vi "execute log.vi"(1 "log window":string, 2 "input string":string) -> (0 "output string":string)   [LabVIEW 2018]
panel:
  out "date/time string":string
  out "current time":timestamp
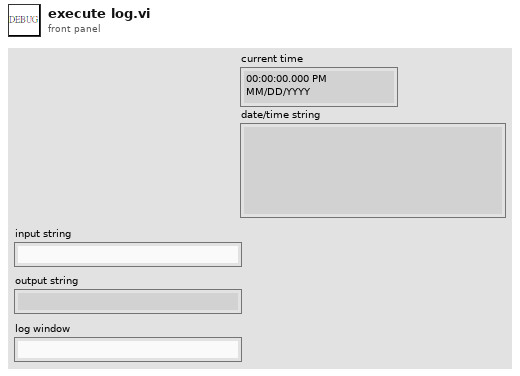
[diagram p1: front panel]
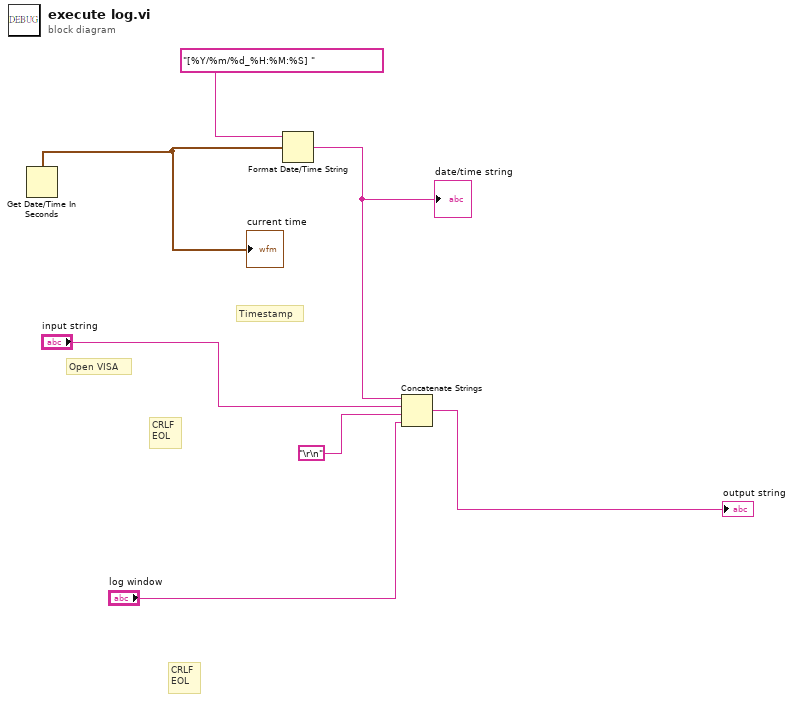
[diagram p0: block diagram]
diagram:
  # "CRLF\nEOL"
  # "CRLF\nEOL"
  # "Timestamp"
  # "Open VISA"
  n1 = Get Date/Time In Seconds() -> (seconds since 1Jan1904=w4:timestamp)
  "current time" <- w4
  n2 = Format Date/Time String(time format string (%c)="[%Y/%m/%d_%H:%M:%S] ", seconds (now)=w4) -> (date/time string=w3:string)  [unwired: 1 in]
  "date/time string" <- w3
  n3 = Concatenate Strings "Concatenate Strings"(w3, "input string", "\r\n", "log window") -> (→"output string":string)
